vi "输入数据解析.vi"(0 "单个参数补充":dbl, 1 "从板号":dbl=1.0, 2 "主板二维码":string="BNET01", 3 "从板二维码":string="BNET01", 5 "主板引用":refnum<vi>, 7 "从板引用":refnum<vi>, 9 "主板选项":string="三级故障阀值", 11 "枚举":enum16{"主板", "从板"}(ring), 12 "快换":bool caption="快换写入") -> (4 "输出数组":dbl[][](array[numeric]), 6 "数组长度":dbl[](array[numeric]), 8 "循环次数":i32, 10 "命令":u32, 14 "名称":string[](array[string]), 15 "命令序号":u32[](array[numeric]))   [LabVIEW 2013] (continued)
                n1942 = disable-structure shown="启用" {
                  disable-tunnel: [w4961 w4964] -> w4957
                  disable-tunnel: [w4960 w4964] -> w4956
                  disable-tunnel: w4954 -> [w4959 _]
                  frame Disabled {
                    n1943 = Unbundle By Name(w4959) -> ("总电压过低"=w4958:dbl)
                    n1944 = call "输入分辨率计算-EV05.vi"("1字节?"=FALSE, "数值"=w4958, "分辨率"=0.1) -> ("低字节"=w4961:dbl, "高字节1"=w4960:dbl)  [unwired: 2 in, 5 out]
                  }
                  frame Enabled {
                    w4964 = 255 ("高字节1")
                  }
                }
                n1945 = Build Array(w4956, w4957) -> (w4955:i32[])
              }
              frame 2 {
                # "温度过高"
                n1946 = disable-structure shown="启用" {
                  disable-tunnel: [w4971 255 ("高字节1")] -> w4967
                  disable-tunnel: w4965 -> [w4969 _]
                  frame Disabled {
                    n1947 = Unbundle By Name(w4969) -> ("温度过高"=w4968:dbl)
                    n1948 = call "输入分辨率计算-EV05.vi"("1字节?"=TRUE, "数值"=w4968, "偏移量"=-40.0, "分辨率"=1.0) -> ("高字节1"=w4971:dbl)  [unwired: 1 in, 6 out]
                  }
                  frame Enabled {
                  }
                }
                n1949 = Build Array(w4967) -> (w4966:i32[])
              }
              frame 3 {
                # "温度过低"
                n1950 = disable-structure shown="启用" {
                  disable-tunnel: [w4981 255 ("高字节1")] -> w4977
                  disable-tunnel: w4975 -> [w4979 _]
                  frame Disabled {
                    n1951 = Unbundle By Name(w4979) -> ("温度过低"=w4978:dbl)
                    n1952 = call "输入分辨率计算-EV05.vi"("1字节?"=TRUE, "数值"=w4978, "偏移量"=-40.0, "分辨率"=1.0) -> ("高字节1"=w4981:dbl)  [unwired: 1 in, 6 out]
                  }
                  frame Enabled {
                  }
                }
                n1953 = Build Array(w4977) -> (w4976:i32[])
              }
              frame 4 {
                # "整组温度不均衡"
                n1954 = disable-structure shown="启用" {
                  disable-tunnel: [w4991 255 ("高字节1")] -> w4987
                  disable-tunnel: w4985 -> [w4989 _]
                  frame Disabled {
                    n1955 = Unbundle By Name(w4989) -> ("整组温度不均衡"=w4988:dbl)
                    n1956 = call "输入分辨率计算-EV05.vi"("1字节?"=TRUE, "数值"=w4988, "偏移量"=0.0, "分辨率"=1.0) -> ("高字节1"=w4991:dbl)  [unwired: 1 in, 6 out]
                  }
                  frame Enabled {
                  }
                }
                n1957 = Build Array(w4987) -> (w4986:i32[])
              }
              frame 5 {
                # "单组电压不均衡"
                n1958 = disable-structure shown="启用" {
                  disable-tunnel: [w5003 w5006] -> w4998
                  disable-tunnel: [w5001 w5006] -> w4996
                  disable-tunnel: w4995 -> [w5000 _]
                  frame Enabled {
                    n1959 = Unbundle By Name(w5000) -> ("单组电压不均衡"=w4999:dbl)
                    n1960 = call "输入分辨率计算-EV05.vi"("1字节?"=FALSE, "数值"=w4999, "偏移量"=0.0, "分辨率"=0.001) -> ("低字节"=w5001:dbl, "高字节1"=w5003:dbl)  [unwired: 1 in, 5 out]
                  }
                  frame Disabled {
                    w5006 = 255 ("高字节1")
                  }
                }
                n1961 = Build Array(w4998, w4996) -> (w4997:dbl[])
              }
              frame 6 {
                # "整组电压不均衡"
                n1962 = disable-structure shown="启用" {
                  disable-tunnel: [w5015 w5018] -> w5010
                  disable-tunnel: [w5013 w5018] -> w5008
                  disable-tunnel: w5007 -> [w5012 _]
                  frame Disabled {
                    n1963 = Unbundle By Name(w5012) -> ("整组电压不均衡"=w5011:dbl)
                    n1964 = call "输入分辨率计算-EV05.vi"("1字节?"=FALSE, "数值"=w5011, "偏移量"=0.0, "分辨率"=0.001) -> ("低字节"=w5013:dbl, "高字节1"=w5015:dbl)  [unwired: 1 in, 5 out]
                  }
                  frame Enabled {
                    w5018 = 255 ("高字节1")
                  }
                }
                n1965 = Build Array(w5010, w5008) -> (w5009:i32[])
              }
              frame 7 {
                # "单体电压过高"
                n1966 = disable-structure shown="启用" {
                  disable-tunnel: [w5027 w5030] -> w5022
                  disable-tunnel: [w5025 w5030] -> w5020
                  disable-tunnel: w5019 -> [w5024 _]
                  frame Disabled {
                    n1967 = Unbundle By Name(w5024) -> ("单体电压过高"=w5023:dbl)
                    n1968 = call "输入分辨率计算-EV05.vi"("1字节?"=FALSE, "数值"=w5023, "偏移量"=0.0, "分辨率"=0.001) -> ("低字节"=w5025:dbl, "高字节1"=w5027:dbl)  [unwired: 1 in, 5 out]
                  }
                  frame Enabled {
                    w5030 = 255 ("高字节1")
                  }
                }
                n1969 = Build Array(w5022, w5020) -> (w5021:i32[])
              }
              frame 8 {
                # "单体电压过低"
                n1970 = disable-structure shown="启用" {
                  disable-tunnel: [w5039 w5042] -> w5034
                  disable-tunnel: [w5037 w5042] -> w5032
                  disable-tunnel: w5031 -> [w5036 _]
                  frame Disabled {
                    n1971 = Unbundle By Name(w5036) -> ("单体电压过低"=w5035:dbl)
                    n1972 = call "输入分辨率计算-EV05.vi"("1字节?"=FALSE, "数值"=w5035, "偏移量"=0.0, "分辨率"=0.001) -> ("低字节"=w5037:dbl, "高字节1"=w5039:dbl)  [unwired: 1 in, 5 out]
                  }
                  frame Enabled {
                    w5042 = 255 ("高字节1")
                  }
                }
                n1973 = Build Array(w5034, w5032) -> (w5033:i32[])
              }
              frame 9 {
                # "充电电流过高"
                n1974 = disable-structure shown="启用" {
                  disable-tunnel: [w5051 w5054] -> w5046
                  disable-tunnel: [w5049 w5054] -> w5044
                  disable-tunnel: w5043 -> [w5048 _]
                  frame Disabled {
                    n1975 = Unbundle By Name(w5048) -> ("充电电流过高"=w5047:dbl)
                    n1976 = call "输入分辨率计算-EV05.vi"("1字节?"=FALSE, "数值"=w5047, "偏移量"=-3000.0, "分辨率"=0.1) -> ("低字节"=w5049:dbl, "高字节1"=w5051:dbl)  [unwired: 1 in, 5 out]
                  }
                  frame Enabled {
                    w5054 = 255 ("高字节1")
                  }
                }
                n1977 = Build Array(w5046, w5044) -> (w5045:i32[])
              }
              frame 10 {
                # "放电电流过高"
                n1978 = disable-structure shown="启用" {
                  disable-tunnel: [w5063 w5066] -> w5058
                  disable-tunnel: [w5061 w5066] -> w5056
                  disable-tunnel: w5055 -> [w5060 _]
                  frame Disabled {
                    n1979 = Unbundle By Name(w5060) -> ("放电电流过高"=w5059:dbl)
                    n1980 = call "输入分辨率计算-EV05.vi"("1字节?"=FALSE, "数值"=w5059, "偏移量"=-3000.0, "分辨率"=0.1) -> ("低字节"=w5061:dbl, "高字节1"=w5063:dbl)  [unwired: 1 in, 5 out]
                  }
                  frame Enabled {
                    w5066 = 255 ("高字节1")
                  }
                }
                n1981 = Build Array(w5058, w5056) -> (w5057:i32[])
              }
              frame 11 {
                # "单组温度不均衡"
                n1982 = disable-structure shown="启用" {
                  disable-tunnel: [w5073 255 ("高字节1")] -> w5069
                  disable-tunnel: w5067 -> [w5071 _]
                  frame Disabled {
                    n1983 = Unbundle By Name(w5071) -> ("单组温度不均衡"=w5070:dbl)
                    n1984 = call "输入分辨率计算-EV05.vi"("1字节?"=TRUE, "数值"=w5070, "偏移量"=0.0, "分辨率"=1.0) -> ("高字节1"=w5073:dbl)  [unwired: 1 in, 6 out]
                  }
                  frame Enabled {
                  }
                }
                n1985 = Build Array(w5069) -> (w5068:i32[])
              }
              frame 12 {
                # "SOC过高"
                n1986 = Unbundle By Name(w5081) -> ("SOC过高"=w5080:dbl)
                n1987 = call "输入分辨率计算-EV05.vi"("1字节?"=FALSE, "数值"=w5080, "偏移量"=0.0, "分辨率"=0.1) -> ("低字节"=w5082:dbl, "高字节1"=w5083:dbl)  [unwired: 1 in, 5 out]
                n1988 = call "二进制解析-8.6.vi"("索引"=4, "数值"=w5083) -> ("低位子数组"=w5086:i32[])  [unwired: 3 out]
                n1989 = call "二进制解析-8.6.vi"("索引"=4, "数值"=w5082) -> ("低位子数组"=w5078:i32[], "高位子数组"=w5085:i32[])  [unwired: 2 out]
                n1990 = Insert Into Array(array=w5086, new element=w5085) -> (w5084:i32[])  [unwired: 1 in]
                n1991 = call "数值二进制转十进制-8.6.vi"("子数组"=w5084) -> ("十进制数值"=w5079:i32)  [unwired: 4 out]
                n1992 = disable-structure shown="启用" {
                  disable-tunnel: w5079 -> [w5094 _]
                  disable-tunnel: [w5094 255 ("高字节1")] -> w5077
                  disable-tunnel: [w5093 i32[] [] ("低位子数组 23")] -> _
                  disable-tunnel: w5078 -> [w5093 _]
                  frame Disabled {
                  }
                  frame Enabled {
                  }
                }
                n1993 = Build Array(w5077, w5077) -> (w5090:i32[])
              }
              frame 13 {
                # "SOC过低"
                n1994 = Unbundle By Name(w5103) -> ("SOC过低"=w5102:dbl)
                n1995 = call "输入分辨率计算-EV05.vi"("1字节?"=FALSE, "数值"=w5102, "偏移量"=0.0, "分辨率"=0.1) -> ("低字节"=w5100:dbl, "高字节1"=w5101:dbl)  [unwired: 1 in, 5 out]
                n1996 = call "二进制解析-8.6.vi"("索引"=4, "数值"=w5101) -> ("低位子数组"=w5098:i32[])  [unwired: 3 out]
                n1997 = disable-structure shown="启用" {
                  disable-tunnel: w5100 -> [w5110 _]
                  disable-tunnel: [w5110 255 ("高字节1")] -> w5099
                  disable-tunnel: w5098 -> [w5109 _]
                  disable-tunnel: [_ 255 ("高字节1")] -> w5097
                  frame Disabled {
                    (unwired) i32[] [] ("低位子数组 4")
                  }
                  frame Enabled {
                  }
                }
                n1998 = Build Array(w5097, w5099) -> (w5106:i32[])
              }
              frame 14 {
                # "内阻过大"
                n1999 = disable-structure shown="启用" {
                  disable-tunnel: w5115 -> [w5120 _]
                  disable-tunnel: [w5116 255 ("高字节1")] -> w5113
                  frame Disabled {
                    n2000 = Unbundle By Name(w5120) -> ("内阻过大"=w5119:dbl)
                    n2001 = call "输入分辨率计算-EV05.vi"("1字节?"=TRUE, "数值"=w5119, "分辨率"=0.1) -> ("高字节1"=w5116:dbl)  [unwired: 2 in, 6 out]
                  }
                  frame Enabled {
                  }
                }
                n2002 = Build Array(w5113) -> (w5114:i32[])
              }
              frame 15 {
                # "极柱温度过高"
                n2003 = disable-structure shown="启用" {
                  disable-tunnel: w5124 -> [w5130 _]
                  disable-tunnel: [w5126 255 ("高字节1")] -> w5122
                  frame Disabled {
                    n2004 = Unbundle By Name(w5130) -> ("极柱温度过高"=w5129:dbl)
                    n2005 = call "输入分辨率计算-EV05.vi"("1字节?"=TRUE, "数值"=w5129, "偏移量"=-40.0, "分辨率"=1.0) -> ("高字节1"=w5126:dbl)  [unwired: 1 in, 6 out]
                  }
                  frame Enabled {
                  }
                }
                n2006 = Build Array(w5122) -> (w5123:i32[])
              }
              frame 16 {
                # "SOH过低"
                n2007 = disable-structure shown="启用" {
                  disable-tunnel: [w5147 w5155] -> w5134
                  disable-tunnel: w5133 -> [w5144 _]
                  disable-tunnel: [w5136 w5155] -> w5132
                  frame Disabled {
                    n2008 = Unbundle By Name(w5144) -> ("SOH过低"=w5143:dbl)
                    n2009 = call "输入分辨率计算-EV05.vi"("1字节?"=FALSE, "数值"=w5143, "偏移量"=0.0, "分辨率"=0.1) -> ("低字节"=w5145:dbl, "高字节1"=w5146:dbl)  [unwired: 1 in, 5 out]
                    n2010 = call "二进制解析-8.6.vi"("索引"=4, "数值"=w5146) -> ("低位子数组"=w5149:i32[])  [unwired: 3 out]
                    n2011 = call "二进制解析-8.6.vi"("索引"=4, "数值"=w5145) -> ("低位子数组"=w5138:i32[], "高位子数组"=w5148:i32[])  [unwired: 2 out]
                    n2012 = call "二进制解析-8.6.vi"("索引"=4, "数值"=0) -> ("低位子数组"=w5139:i32[])  [unwired: 3 out]
                    n2013 = Insert Into Array(array=w5149, new element=w5148) -> (w5142:i32[])  [unwired: 1 in]
                    n2014 = Insert Into Array(array=w5138, new element=w5139) -> (w5137:i32[])  [unwired: 1 in]
                    n2015 = call "数值二进制转十进制-8.6.vi"("子数组"=w5142) -> ("十进制数值"=w5147:i32)  [unwired: 4 out]
                    n2016 = call "数值二进制转十进制-8.6.vi"("子数组"=w5137) -> ("十进制数值"=w5136:i32)  [unwired: 4 out]
                  }
                  frame Enabled {
                    w5155 = 255 ("高字节1")
                  }
                }
                n2017 = Build Array(w5134, w5132) -> (w5135:i32[])
              }
            }
            n2018 = Insert Into Array(array=w4939, new element=w4940) -> (w4938:dbl[])  [unwired: 1 in]
          }
          n2019 = Build Array(w4935) -> (w4934:dbl[][])
          n2020 = Build Array("三级故障阀值") -> (w4925:string[])
        }
        frame "整组电压不均衡" {
          n2021 = Unbundle By Name(w5161) -> ("一级故障"=w5162:refnum<vi>)
          n2022 = property class="Clust (严格)"(reference=w5162) -> ("Value"=w5160:T4)  [unwired: 1 in, 2 out]
          n2023 = for {
            N: 17 -> [_]
            tunnel: w5160 -> [w5172]
            shift-right: [w5169] -> w5166
            shift-left: dbl[] [] -> [w5170]
            i -> [w5173]
            n2024 = case shown="13" w5173 {
              tunnel: w5172 -> [w5174 w5185 w5196 w5206 w5216 w5226 w5238 w5250 w5262 w5274 w5286 w5298 w5312 w5333 w5344 w5353 w5362]
              tunnel: [w5175 w5186 w5197 w5207 w5217 w5228 w5240 w5252 w5264 w5276 w5288 w5299 w5321 w5336 w5343 w5352 w5364] -> w5171
              frame 0, Default {
                # "总电压过高"
                n2025 = disable-structure shown="启用" {
                  disable-tunnel: [w5181 w5184] -> w5177
                  disable-tunnel: [w5180 w5184] -> w5176
                  disable-tunnel: w5174 -> [w5179 _]
                  frame Disabled {
                    n2026 = Unbundle By Name(w5179) -> ("总电压过高"=w5178:dbl)
                    n2027 = call "输入分辨率计算-EV05.vi"("1字节?"=FALSE, "数值"=w5178, "分辨率"=0.1) -> ("低字节"=w5181:dbl, "高字节1"=w5180:dbl)  [unwired: 2 in, 5 out]
                  }
                  frame Enabled {
                    w5184 = 255 ("高字节1")
                  }
                }
                n2028 = Build Array(w5176, w5177) -> (w5175:i32[])
              }
              frame 1 {
                # "总电压过低"
                n2029 = disable-structure shown="启用" {
                  disable-tunnel: [w5192 w5195] -> w5188
                  disable-tunnel: [w5191 w5195] -> w5187
                  disable-tunnel: w5185 -> [w5190 _]
                  frame Disabled {
                    n2030 = Unbundle By Name(w5190) -> ("总电压过低"=w5189:dbl)
                    n2031 = call "输入分辨率计算-EV05.vi"("1字节?"=FALSE, "数值"=w5189, "分辨率"=0.1) -> ("低字节"=w5192:dbl, "高字节1"=w5191:dbl)  [unwired: 2 in, 5 out]
                  }
                  frame Enabled {
                    w5195 = 255 ("高字节1")
                  }
                }
                n2032 = Build Array(w5187, w5188) -> (w5186:i32[])
              }
              frame 2 {
                # "温度过高"
                n2033 = disable-structure shown="启用" {
                  disable-tunnel: [w5202 255 ("高字节1")] -> w5198
                  disable-tunnel: w5196 -> [w5200 _]
                  frame Disabled {
                    n2034 = Unbundle By Name(w5200) -> ("温度过高"=w5199:dbl)
                    n2035 = call "输入分辨率计算-EV05.vi"("1字节?"=TRUE, "数值"=w5199, "偏移量"=-40.0, "分辨率"=1.0) -> ("高字节1"=w5202:dbl)  [unwired: 1 in, 6 out]
                  }
                  frame Enabled {
                  }
                }
                n2036 = Build Array(w5198) -> (w5197:i32[])
              }
              frame 3 {
                # "温度过低"
                n2037 = disable-structure shown="启用" {
                  disable-tunnel: [w5212 255 ("高字节1")] -> w5208
                  disable-tunnel: w5206 -> [w5210 _]
                  frame Disabled {
                    n2038 = Unbundle By Name(w5210) -> ("温度过低"=w5209:dbl)
                    n2039 = call "输入分辨率计算-EV05.vi"("1字节?"=TRUE, "数值"=w5209, "偏移量"=-40.0, "分辨率"=1.0) -> ("高字节1"=w5212:dbl)  [unwired: 1 in, 6 out]
                  }
                  frame Enabled {
                  }
                }
                n2040 = Build Array(w5208) -> (w5207:i32[])
              }
              frame 4 {
                # "整组温度不均衡"
                n2041 = disable-structure shown="启用" {
                  disable-tunnel: [w5222 255 ("高字节1")] -> w5218
                  disable-tunnel: w5216 -> [w5220 _]
                  frame Disabled {
                    n2042 = Unbundle By Name(w5220) -> ("整组温度不均衡"=w5219:dbl)
                    n2043 = call "输入分辨率计算-EV05.vi"("1字节?"=TRUE, "数值"=w5219, "偏移量"=0.0, "分辨率"=1.0) -> ("高字节1"=w5222:dbl)  [unwired: 1 in, 6 out]
                  }
                  frame Enabled {
                  }
                }
                n2044 = Build Array(w5218) -> (w5217:i32[])
              }
              frame 5 {
                # "单组电压不均衡"
                n2045 = disable-structure shown="启用" {
                  disable-tunnel: [w5234 w5237] -> w5229
                  disable-tunnel: [w5232 w5237] -> w5227
                  disable-tunnel: w5226 -> [w5231 _]
                  frame Disabled {
                    n2046 = Unbundle By Name(w5231) -> ("单组电压不均衡"=w5230:dbl)
                    n2047 = call "输入分辨率计算-EV05.vi"("1字节?"=FALSE, "数值"=w5230, "偏移量"=0.0, "分辨率"=0.001) -> ("低字节"=w5232:dbl, "高字节1"=w5234:dbl)  [unwired: 1 in, 5 out]
                  }
                  frame Enabled {
                    w5237 = 255 ("高字节1")
                  }
                }
                n2048 = Build Array(w5229, w5227) -> (w5228:i32[])
              }
              frame 6 {
                # "整组电压不均衡"
                n2049 = disable-structure shown="启用" {
                  disable-tunnel: [w5246 w5249] -> w5241
                  disable-tunnel: [w5244 w5249] -> w5239
                  disable-tunnel: w5238 -> [w5243 _]
                  frame Enabled {
                    n2050 = Unbundle By Name(w5243) -> ("整组电压不均衡"=w5242:dbl)
                    n2051 = call "输入分辨率计算-EV05.vi"("1字节?"=FALSE, "数值"=w5242, "偏移量"=0.0, "分辨率"=0.001) -> ("低字节"=w5244:dbl, "高字节1"=w5246:dbl)  [unwired: 1 in, 5 out]
                  }
                  frame Disabled {
                    w5249 = 255 ("高字节1")
                  }
                }
                n2052 = Build Array(w5241, w5239) -> (w5240:dbl[])
              }
              frame 7 {
                # "单体电压过高"
                n2053 = disable-structure shown="启用" {
                  disable-tunnel: [w5258 w5261] -> w5253
                  disable-tunnel: [w5256 w5261] -> w5251
                  disable-tunnel: w5250 -> [w5255 _]
                  frame Disabled {
                    n2054 = Unbundle By Name(w5255) -> ("单体电压过高"=w5254:dbl)
                    n2055 = call "输入分辨率计算-EV05.vi"("1字节?"=FALSE, "数值"=w5254, "偏移量"=0.0, "分辨率"=0.001) -> ("低字节"=w5256:dbl, "高字节1"=w5258:dbl)  [unwired: 1 in, 5 out]
                  }
                  frame Enabled {
                    w5261 = 255 ("高字节1")
                  }
                }
                n2056 = Build Array(w5253, w5251) -> (w5252:i32[])
              }
              frame 8 {
                # "单体电压过低"
                n2057 = disable-structure shown="启用" {
                  disable-tunnel: [w5270 w5273] -> w5265
                  disable-tunnel: [w5268 w5273] -> w5263
                  disable-tunnel: w5262 -> [w5267 _]
                  frame Disabled {
                    n2058 = Unbundle By Name(w5267) -> ("单体电压过低"=w5266:dbl)
                    n2059 = call "输入分辨率计算-EV05.vi"("1字节?"=FALSE, "数值"=w5266, "偏移量"=0.0, "分辨率"=0.001) -> ("低字节"=w5268:dbl, "高字节1"=w5270:dbl)  [unwired: 1 in, 5 out]
                  }
                  frame Enabled {
                    w5273 = 255 ("高字节1")
                  }
                }
                n2060 = Build Array(w5265, w5263) -> (w5264:i32[])
              }
              frame 9 {
                # "充电电流过高"
                n2061 = disable-structure shown="启用" {
                  disable-tunnel: [w5282 w5285] -> w5277
                  disable-tunnel: [w5280 w5285] -> w5275
                  disable-tunnel: w5274 -> [w5279 _]
                  frame Disabled {
                    n2062 = Unbundle By Name(w5279) -> ("充电电流过高"=w5278:dbl)
                    n2063 = call "输入分辨率计算-EV05.vi"("1字节?"=FALSE, "数值"=w5278, "偏移量"=-3000.0, "分辨率"=0.1) -> ("低字节"=w5280:dbl, "高字节1"=w5282:dbl)  [unwired: 1 in, 5 out]
                  }
                  frame Enabled {
                    w5285 = 255 ("高字节1")
                  }
                }
                n2064 = Build Array(w5277, w5275) -> (w5276:i32[])
              }
              frame 10 {
                # "放电电流过高"
                n2065 = disable-structure shown="启用" {
                  disable-tunnel: [w5294 w5297] -> w5289
                  disable-tunnel: [w5292 w5297] -> w5287
                  disable-tunnel: w5286 -> [w5291 _]
                  frame Disabled {
                    n2066 = Unbundle By Name(w5291) -> ("放电电流过高"=w5290:dbl)
                    n2067 = call "输入分辨率计算-EV05.vi"("1字节?"=FALSE, "数值"=w5290, "偏移量"=-3000.0, "分辨率"=0.1) -> ("低字节"=w5292:dbl, "高字节1"=w5294:dbl)  [unwired: 1 in, 5 out]
                  }
                  frame Enabled {
                    w5297 = 255 ("高字节1")
                  }
                }
                n2068 = Build Array(w5289, w5287) -> (w5288:i32[])
              }
              frame 11 {
                # "单组温度不均衡"
                n2069 = disable-structure shown="启用" {
                  disable-tunnel: [w5304 255 ("高字节1")] -> w5300
                  disable-tunnel: w5298 -> [w5302 _]
                  frame Disabled {
                    n2070 = Unbundle By Name(w5302) -> ("单组温度不均衡"=w5301:dbl)
                    n2071 = call "输入分辨率计算-EV05.vi"("1字节?"=TRUE, "数值"=w5301, "偏移量"=0.0, "分辨率"=1.0) -> ("高字节1"=w5304:dbl)  [unwired: 1 in, 6 out]
                  }
                  frame Enabled {
                  }
                }
                n2072 = Build Array(w5300) -> (w5299:i32[])
              }
              frame 12 {
                # "SOC过高"
                n2073 = Unbundle By Name(w5312) -> ("SOC过高"=w5311:dbl)
                n2074 = call "输入分辨率计算-EV05.vi"("1字节?"=FALSE, "数值"=w5311, "偏移量"=0.0, "分辨率"=0.1) -> ("低字节"=w5313:dbl, "高字节1"=w5314:dbl)  [unwired: 1 in, 5 out]
                n2075 = call "二进制解析-8.6.vi"("索引"=4, "数值"=w5314) -> ("低位子数组"=w5317:i32[])  [unwired: 3 out]
                n2076 = call "二进制解析-8.6.vi"("索引"=4, "数值"=w5313) -> ("低位子数组"=w5309:i32[], "高位子数组"=w5316:i32[])  [unwired: 2 out]
                n2077 = Insert Into Array(array=w5317, new element=w5316) -> (w5315:i32[])  [unwired: 1 in]
                n2078 = call "数值二进制转十进制-8.6.vi"("子数组"=w5315) -> ("十进制数值"=w5310:i32)  [unwired: 4 out]
                n2079 = disable-structure shown="启用" {
                  disable-tunnel: w5310 -> [w5325 _]
                  disable-tunnel: [w5325 255 ("高字节1")] -> w5308
                  disable-tunnel: [w5324 i32[] [] ("低位子数组 24")] -> _
                  disable-tunnel: w5309 -> [w5324 _]
                  frame Disabled {
                  }
                  frame Enabled {
                  }
                }
                n2080 = Build Array(w5308, w5308) -> (w5321:i32[])
              }
              frame 13 {
                # "SOC过低"
                n2081 = Unbundle By Name(w5333) -> ("SOC过低"=w5332:dbl)
                n2082 = call "输入分辨率计算-EV05.vi"("1字节?"=FALSE, "数值"=w5332, "偏移量"=0.0, "分辨率"=0.1) -> ("低字节"=w5330:dbl, "高字节1"=w5331:dbl)  [unwired: 1 in, 5 out]
                n2083 = call "二进制解析-8.6.vi"("索引"=4, "数值"=w5331) -> ("低位子数组"=w5329:i32[])  [unwired: 3 out]
                n2084 = disable-structure shown="启用" {
                  disable-tunnel: w5330 -> [w5340 _]
                  disable-tunnel: [w5340 255 ("高字节1")] -> w5328
                  disable-tunnel: w5329 -> [w5339 _]
                  frame Disabled {
                    (unwired) i32[] [] ("低位子数组 4")
                  }
                  frame Enabled {
                  }
                }
                n2085 = Build Array(w5328, w5328) -> (w5336:i32[])
              }
              frame 14 {
                # "内阻过大"
                n2086 = disable-structure shown="启用" {
                  disable-tunnel: w5344 -> [w5349 _]
                  disable-tunnel: [w5345 255 ("高字节1")] -> w5342
                  frame Disabled {
                    n2087 = Unbundle By Name(w5349) -> ("内阻过大"=w5348:dbl)
                    n2088 = call "输入分辨率计算-EV05.vi"("1字节?"=TRUE, "数值"=w5348, "分辨率"=0.1) -> ("高字节1"=w5345:dbl)  [unwired: 2 in, 6 out]
                  }
                  frame Enabled {
                  }
                }
                n2089 = Build Array(w5342) -> (w5343:i32[])
              }
              frame 15 {
                # "极柱温度过高"
                n2090 = disable-structure shown="启用" {
                  disable-tunnel: w5353 -> [w5359 _]
                  disable-tunnel: [w5355 255 ("高字节1")] -> w5351
                  frame Disabled {
                    n2091 = Unbundle By Name(w5359) -> ("极柱温度过高"=w5358:dbl)
                    n2092 = call "输入分辨率计算-EV05.vi"("1字节?"=TRUE, "数值"=w5358, "偏移量"=-40.0, "分辨率"=1.0) -> ("高字节1"=w5355:dbl)  [unwired: 1 in, 6 out]
                  }
                  frame Enabled {
                  }
                }
                n2093 = Build Array(w5351) -> (w5352:i32[])
              }
              frame 16 {
                # "SOH过低"
                n2094 = disable-structure shown="启用" {
                  disable-tunnel: [w5376 w5384] -> w5363
                  disable-tunnel: w5362 -> [w5373 _]
                  disable-tunnel: [w5365 w5384] -> w5361
                  frame Disabled {
                    n2095 = Unbundle By Name(w5373) -> ("SOH过低"=w5372:dbl)
                    n2096 = call "输入分辨率计算-EV05.vi"("1字节?"=FALSE, "数值"=w5372, "偏移量"=0.0, "分辨率"=0.1) -> ("低字节"=w5374:dbl, "高字节1"=w5375:dbl)  [unwired: 1 in, 5 out]
                    n2097 = call "二进制解析-8.6.vi"("索引"=4, "数值"=w5375) -> ("低位子数组"=w5378:i32[])  [unwired: 3 out]
                    n2098 = call "二进制解析-8.6.vi"("索引"=4, "数值"=w5374) -> ("低位子数组"=w5367:i32[], "高位子数组"=w5377:i32[])  [unwired: 2 out]
                    n2099 = call "二进制解析-8.6.vi"("索引"=4, "数值"=0) -> ("低位子数组"=w5368:i32[])  [unwired: 3 out]
                    n2100 = Insert Into Array(array=w5378, new element=w5377) -> (w5371:i32[])  [unwired: 1 in]
                    n2101 = Insert Into Array(array=w5367, new element=w5368) -> (w5366:i32[])  [unwired: 1 in]
                    n2102 = call "数值二进制转十进制-8.6.vi"("子数组"=w5371) -> ("十进制数值"=w5376:i32)  [unwired: 4 out]
                    n2103 = call "数值二进制转十进制-8.6.vi"("子数组"=w5366) -> ("十进制数值"=w5365:i32)  [unwired: 4 out]
                  }
                  frame Enabled {
                    w5384 = 255 ("高字节1")
                  }
                }
                n2104 = Build Array(w5363, w5361) -> (w5364:i32[])
              }
            }
            n2105 = Insert Into Array(array=w5170, new element=w5171) -> (w5169:dbl[])  [unwired: 1 in]
          }
          n2106 = Build Array(w5166) -> (w5165:dbl[][])
          n2107 = Build Array("一级故障阀值") -> (w5156:string[])
        }
        frame "整组电压不均衡(2)" {
          n2108 = Unbundle By Name(w5390) -> ("一级故障 2"=w5391:refnum<vi>)
          n2109 = property class="Clust (严格)"(reference=w5391) -> ("Value"=w5389:T4)  [unwired: 1 in, 2 out]
          n2110 = for {
            N: 17 -> [_]
            tunnel: w5389 -> [w5401]
            shift-right: [w5398] -> w5395
            shift-left: dbl[] [] -> [w5399]
            i -> [w5402]
            n2111 = case shown="13" w5402 {
              tunnel: w5401 -> [w5403 w5414 w5425 w5435 w5445 w5455 w5467 w5479 w5491 w5503 w5515 w5527 w5541 w5562 w5573 w5582 w5591]
              tunnel: [w5404 w5415 w5426 w5436 w5446 w5457 w5469 w5481 w5493 w5505 w5517 w5528 w5550 w5565 w5572 w5581 w5593] -> w5400
              frame 0, Default {
                # "总电压过高"
                n2112 = disable-structure shown="启用" {
                  disable-tunnel: [w5410 w5413] -> w5406
                  disable-tunnel: [w5409 w5413] -> w5405
                  disable-tunnel: w5403 -> [w5408 _]
                  frame Disabled {
                    n2113 = Unbundle By Name(w5408) -> ("总电压过高"=w5407:dbl)
                    n2114 = call "输入分辨率计算-EV05.vi"("1字节?"=FALSE, "数值"=w5407, "分辨率"=0.1) -> ("低字节"=w5410:dbl, "高字节1"=w5409:dbl)  [unwired: 2 in, 5 out]
                  }
                  frame Enabled {
                    w5413 = 255 ("高字节1")
                  }
                }
                n2115 = Build Array(w5405, w5406) -> (w5404:i32[])
              }
              frame 1 {
                # "总电压过低"
                n2116 = disable-structure shown="启用" {
                  disable-tunnel: [w5421 w5424] -> w5417
                  disable-tunnel: [w5420 w5424] -> w5416
                  disable-tunnel: w5414 -> [w5419 _]
                  frame Disabled {
                    n2117 = Unbundle By Name(w5419) -> ("总电压过低"=w5418:dbl)
                    n2118 = call "输入分辨率计算-EV05.vi"("1字节?"=FALSE, "数值"=w5418, "分辨率"=0.1) -> ("低字节"=w5421:dbl, "高字节1"=w5420:dbl)  [unwired: 2 in, 5 out]
                  }
                  frame Enabled {
                    w5424 = 255 ("高字节1")
                  }
                }
                n2119 = Build Array(w5416, w5417) -> (w5415:i32[])
              }
              frame 2 {
                # "温度过高"
                n2120 = disable-structure shown="启用" {
                  disable-tunnel: [w5431 255 ("高字节1")] -> w5427
                  disable-tunnel: w5425 -> [w5429 _]
                  frame Disabled {
                    n2121 = Unbundle By Name(w5429) -> ("温度过高"=w5428:dbl)
                    n2122 = call "输入分辨率计算-EV05.vi"("1字节?"=TRUE, "数值"=w5428, "偏移量"=-40.0, "分辨率"=1.0) -> ("高字节1"=w5431:dbl)  [unwired: 1 in, 6 out]
                  }
                  frame Enabled {
                  }
                }
                n2123 = Build Array(w5427) -> (w5426:i32[])
              }
              frame 3 {
                # "温度过低"
                n2124 = disable-structure shown="启用" {
                  disable-tunnel: [w5441 255 ("高字节1")] -> w5437
                  disable-tunnel: w5435 -> [w5439 _]
                  frame Disabled {
                    n2125 = Unbundle By Name(w5439) -> ("温度过低"=w5438:dbl)
                    n2126 = call "输入分辨率计算-EV05.vi"("1字节?"=TRUE, "数值"=w5438, "偏移量"=-40.0, "分辨率"=1.0) -> ("高字节1"=w5441:dbl)  [unwired: 1 in, 6 out]
                  }
                  frame Enabled {
                  }
                }
                n2127 = Build Array(w5437) -> (w5436:i32[])
              }
              frame 4 {
                # "整组温度不均衡"
                n2128 = disable-structure shown="启用" {
                  disable-tunnel: [w5451 255 ("高字节1")] -> w5447
                  disable-tunnel: w5445 -> [w5449 _]
                  frame Disabled {
                    n2129 = Unbundle By Name(w5449) -> ("整组温度不均衡"=w5448:dbl)
                    n2130 = call "输入分辨率计算-EV05.vi"("1字节?"=TRUE, "数值"=w5448, "偏移量"=0.0, "分辨率"=1.0) -> ("高字节1"=w5451:dbl)  [unwired: 1 in, 6 out]
                  }
                  frame Enabled {
                  }
                }
                n2131 = Build Array(w5447) -> (w5446:i32[])
              }
              frame 5 {
                # "单组电压不均衡"
                n2132 = disable-structure shown="启用" {
                  disable-tunnel: [w5463 w5466] -> w5458
                  disable-tunnel: [w5461 w5466] -> w5456
                  disable-tunnel: w5455 -> [w5460 _]
                  frame Disabled {
                    n2133 = Unbundle By Name(w5460) -> ("单组电压不均衡"=w5459:dbl)
                    n2134 = call "输入分辨率计算-EV05.vi"("1字节?"=FALSE, "数值"=w5459, "偏移量"=0.0, "分辨率"=0.001) -> ("低字节"=w5461:dbl, "高字节1"=w5463:dbl)  [unwired: 1 in, 5 out]
                  }
                  frame Enabled {
                    w5466 = 255 ("高字节1")
                  }
                }
                n2135 = Build Array(w5458, w5456) -> (w5457:i32[])
              }
              frame 6 {
                # "整组电压不均衡"
                n2136 = disable-structure shown="启用" {
                  disable-tunnel: [w5475 w5478] -> w5470
                  disable-tunnel: [w5473 w5478] -> w5468
                  disable-tunnel: w5467 -> [w5472 _]
                  frame Enabled {
                    n2137 = Unbundle By Name(w5472) -> ("整组电压不均衡"=w5471:dbl)
                    n2138 = call "输入分辨率计算-EV05.vi"("1字节?"=FALSE, "数值"=w5471, "偏移量"=0.0, "分辨率"=0.001) -> ("低字节"=w5473:dbl, "高字节1"=w5475:dbl)  [unwired: 1 in, 5 out]
                  }
                  frame Disabled {
                    w5478 = 255 ("高字节1")
                  }
                }
                n2139 = Build Array(w5470, w5468) -> (w5469:dbl[])
              }
              frame 7 {
                # "单体电压过高"
                n2140 = disable-structure shown="启用" {
                  disable-tunnel: [w5487 w5490] -> w5482
                  disable-tunnel: [w5485 w5490] -> w5480
                  disable-tunnel: w5479 -> [w5484 _]
                  frame Disabled {
                    n2141 = Unbundle By Name(w5484) -> ("单体电压过高"=w5483:dbl)
                    n2142 = call "输入分辨率计算-EV05.vi"("1字节?"=FALSE, "数值"=w5483, "偏移量"=0.0, "分辨率"=0.001) -> ("低字节"=w5485:dbl, "高字节1"=w5487:dbl)  [unwired: 1 in, 5 out]
                  }
                  frame Enabled {
                    w5490 = 255 ("高字节1")
                  }
                }
                n2143 = Build Array(w5482, w5480) -> (w5481:i32[])
              }
              frame 8 {
                # "单体电压过低"
                n2144 = disable-structure shown="启用" {
                  disable-tunnel: [w5499 w5502] -> w5494
                  disable-tunnel: [w5497 w5502] -> w5492
                  disable-tunnel: w5491 -> [w5496 _]
                  frame Disabled {
                    n2145 = Unbundle By Name(w5496) -> ("单体电压过低"=w5495:dbl)
                    n2146 = call "输入分辨率计算-EV05.vi"("1字节?"=FALSE, "数值"=w5495, "偏移量"=0.0, "分辨率"=0.001) -> ("低字节"=w5497:dbl, "高字节1"=w5499:dbl)  [unwired: 1 in, 5 out]
                  }
                  frame Enabled {
                    w5502 = 255 ("高字节1")
                  }
                }
                n2147 = Build Array(w5494, w5492) -> (w5493:i32[])
              }
              frame 9 {
                # "充电电流过高"
                n2148 = disable-structure shown="启用" {
                  disable-tunnel: [w5511 w5514] -> w5506
                  disable-tunnel: [w5509 w5514] -> w5504
                  disable-tunnel: w5503 -> [w5508 _]
                  frame Disabled {
                    n2149 = Unbundle By Name(w5508) -> ("充电电流过高"=w5507:dbl)
                    n2150 = call "输入分辨率计算-EV05.vi"("1字节?"=FALSE, "数值"=w5507, "偏移量"=-3000.0, "分辨率"=0.1) -> ("低字节"=w5509:dbl, "高字节1"=w5511:dbl)  [unwired: 1 in, 5 out]
                  }
                  frame Enabled {
                    w5514 = 255 ("高字节1")
                  }
                }
                n2151 = Build Array(w5506, w5504) -> (w5505:i32[])
              }
              frame 10 {
                # "放电电流过高"
                n2152 = disable-structure shown="启用" {
                  disable-tunnel: [w5523 w5526] -> w5518
                  disable-tunnel: [w5521 w5526] -> w5516
                  disable-tunnel: w5515 -> [w5520 _]
                  frame Disabled {
                    n2153 = Unbundle By Name(w5520) -> ("放电电流过高"=w5519:dbl)
                    n2154 = call "输入分辨率计算-EV05.vi"("1字节?"=FALSE, "数值"=w5519, "偏移量"=-3000.0, "分辨率"=0.1) -> ("低字节"=w5521:dbl, "高字节1"=w5523:dbl)  [unwired: 1 in, 5 out]
                  }
                  frame Enabled {
                    w5526 = 255 ("高字节1")
                  }
                }
                n2155 = Build Array(w5518, w5516) -> (w5517:i32[])
              }
              frame 11 {
                # "单组温度不均衡"
                n2156 = disable-structure shown="启用" {
                  disable-tunnel: [w5533 255 ("高字节1")] -> w5529
                  disable-tunnel: w5527 -> [w5531 _]
                  frame Disabled {
                    n2157 = Unbundle By Name(w5531) -> ("单组温度不均衡"=w5530:dbl)
                    n2158 = call "输入分辨率计算-EV05.vi"("1字节?"=TRUE, "数值"=w5530, "偏移量"=0.0, "分辨率"=1.0) -> ("高字节1"=w5533:dbl)  [unwired: 1 in, 6 out]
                  }
                  frame Enabled {
                  }
                }
                n2159 = Build Array(w5529) -> (w5528:i32[])
              }
              frame 12 {
                # "SOC过高"
                n2160 = Unbundle By Name(w5541) -> ("SOC过高"=w5540:dbl)
                n2161 = call "输入分辨率计算-EV05.vi"("1字节?"=FALSE, "数值"=w5540, "偏移量"=0.0, "分辨率"=0.1) -> ("低字节"=w5542:dbl, "高字节1"=w5543:dbl)  [unwired: 1 in, 5 out]
                n2162 = call "二进制解析-8.6.vi"("索引"=4, "数值"=w5543) -> ("低位子数组"=w5546:i32[])  [unwired: 3 out]
                n2163 = call "二进制解析-8.6.vi"("索引"=4, "数值"=w5542) -> ("低位子数组"=w5538:i32[], "高位子数组"=w5545:i32[])  [unwired: 2 out]
                n2164 = Insert Into Array(array=w5546, new element=w5545) -> (w5544:i32[])  [unwired: 1 in]
                n2165 = call "数值二进制转十进制-8.6.vi"("子数组"=w5544) -> ("十进制数值"=w5539:i32)  [unwired: 4 out]
                n2166 = disable-structure shown="启用" {
                  disable-tunnel: w5539 -> [w5554 _]
                  disable-tunnel: [w5554 255 ("高字节1")] -> w5537
                  disable-tunnel: [w5553 i32[] [] ("低位子数组 24")] -> _
                  disable-tunnel: w5538 -> [w5553 _]
                  frame Disabled {
                  }
                  frame Enabled {
                  }
                }
                n2167 = Build Array(w5537, w5537) -> (w5550:i32[])
              }
              frame 13 {
                # "SOC过低"
                n2168 = Unbundle By Name(w5562) -> ("SOC过低"=w5561:dbl)
                n2169 = call "输入分辨率计算-EV05.vi"("1字节?"=FALSE, "数值"=w5561, "偏移量"=0.0, "分辨率"=0.1) -> ("低字节"=w5559:dbl, "高字节1"=w5560:dbl)  [unwired: 1 in, 5 out]
                n2170 = call "二进制解析-8.6.vi"("索引"=4, "数值"=w5560) -> ("低位子数组"=w5558:i32[])  [unwired: 3 out]
                n2171 = disable-structure shown="启用" {
                  disable-tunnel: w5559 -> [w5569 _]
                  disable-tunnel: [w5569 255 ("高字节1")] -> w5557
                  disable-tunnel: w5558 -> [w5568 _]
                  frame Disabled {
                    (unwired) i32[] [] ("低位子数组 4")
                  }
                  frame Enabled {
                  }
                }
                n2172 = Build Array(w5557, w5557) -> (w5565:i32[])
              }
              frame 14 {
                # "内阻过大"
                n2173 = disable-structure shown="启用" {
                  disable-tunnel: w5573 -> [w5578 _]
                  disable-tunnel: [w5574 255 ("高字节1")] -> w5571
                  frame Disabled {
                    n2174 = Unbundle By Name(w5578) -> ("内阻过大"=w5577:dbl)
                    n2175 = call "输入分辨率计算-EV05.vi"("1字节?"=TRUE, "数值"=w5577, "分辨率"=0.1) -> ("高字节1"=w5574:dbl)  [unwired: 2 in, 6 out]
                  }
                  frame Enabled {
                  }
                }
                n2176 = Build Array(w5571) -> (w5572:i32[])
              }
              frame 15 {
                # "极柱温度过高"
                n2177 = disable-structure shown="启用" {
                  disable-tunnel: w5582 -> [w5588 _]
                  disable-tunnel: [w5584 255 ("高字节1")] -> w5580
                  frame Disabled {
                    n2178 = Unbundle By Name(w5588) -> ("极柱温度过高"=w5587:dbl)
                    n2179 = call "输入分辨率计算-EV05.vi"("1字节?"=TRUE, "数值"=w5587, "偏移量"=-40.0, "分辨率"=1.0) -> ("高字节1"=w5584:dbl)  [unwired: 1 in, 6 out]
                  }
                  frame Enabled {
                  }
                }
                n2180 = Build Array(w5580) -> (w5581:i32[])
              }
              frame 16 {
                # "SOH过低"
                n2181 = disable-structure shown="启用" {
                  disable-tunnel: [w5605 w5613] -> w5592
                  disable-tunnel: w5591 -> [w5602 _]
                  disable-tunnel: [w5594 w5613] -> w5590
                  frame Disabled {
                    n2182 = Unbundle By Name(w5602) -> ("SOH过低"=w5601:dbl)
                    n2183 = call "输入分辨率计算-EV05.vi"("1字节?"=FALSE, "数值"=w5601, "偏移量"=0.0, "分辨率"=0.1) -> ("低字节"=w5603:dbl, "高字节1"=w5604:dbl)  [unwired: 1 in, 5 out]
                    n2184 = call "二进制解析-8.6.vi"("索引"=4, "数值"=w5604) -> ("低位子数组"=w5607:i32[])  [unwired: 3 out]
                    n2185 = call "二进制解析-8.6.vi"("索引"=4, "数值"=w5603) -> ("低位子数组"=w5596:i32[], "高位子数组"=w5606:i32[])  [unwired: 2 out]
                    n2186 = call "二进制解析-8.6.vi"("索引"=4, "数值"=0) -> ("低位子数组"=w5597:i32[])  [unwired: 3 out]
                    n2187 = Insert Into Array(array=w5607, new element=w5606) -> (w5600:i32[])  [unwired: 1 in]
                    n2188 = Insert Into Array(array=w5596, new element=w5597) -> (w5595:i32[])  [unwired: 1 in]
                    n2189 = call "数值二进制转十进制-8.6.vi"("子数组"=w5600) -> ("十进制数值"=w5605:i32)  [unwired: 4 out]
                    n2190 = call "数值二进制转十进制-8.6.vi"("子数组"=w5595) -> ("十进制数值"=w5594:i32)  [unwired: 4 out]
                  }
                  frame Enabled {
                    w5613 = 255 ("高字节1")
                  }
                }
                n2191 = Build Array(w5592, w5590) -> (w5593:i32[])
              }
            }
            n2192 = Insert Into Array(array=w5399, new element=w5400) -> (w5398:dbl[])  [unwired: 1 in]
          }
          n2193 = Build Array(w5395) -> (w5394:dbl[][])
          n2194 = Build Array("二级故障阀值") -> (w5385:string[])
        }
        frame "整组电压不均衡(3)" {
          n2195 = Unbundle By Name(w5619) -> ("一级故障 3"=w5620:refnum<vi>)
          n2196 = property class="Clust (严格)"(reference=w5620) -> ("Value"=w5618:T4)  [unwired: 1 in, 2 out]
          n2197 = for {
            N: 17 -> [_]
            tunnel: w5618 -> [w5630]
            shift-right: [w5627] -> w5624
            shift-left: dbl[] [] -> [w5628]
            i -> [w5631]
            n2198 = case shown="13" w5631 {
              tunnel: w5630 -> [w5632 w5643 w5654 w5664 w5674 w5684 w5696 w5708 w5720 w5732 w5744 w5756 w5770 w5791 w5802 w5811 w5820]
              tunnel: [w5633 w5644 w5655 w5665 w5675 w5686 w5698 w5710 w5722 w5734 w5746 w5757 w5779 w5794 w5801 w5810 w5822] -> w5629
              frame 0, Default {
                # "总电压过高"
                n2199 = disable-structure shown="启用" {
                  disable-tunnel: [w5639 w5642] -> w5635
                  disable-tunnel: [w5638 w5642] -> w5634
                  disable-tunnel: w5632 -> [w5637 _]
                  frame Disabled {
                    n2200 = Unbundle By Name(w5637) -> ("总电压过高"=w5636:dbl)
                    n2201 = call "输入分辨率计算-EV05.vi"("1字节?"=FALSE, "数值"=w5636, "分辨率"=0.1) -> ("低字节"=w5639:dbl, "高字节1"=w5638:dbl)  [unwired: 2 in, 5 out]
                  }
                  frame Enabled {
                    w5642 = 255 ("高字节1")
                  }
                }
                n2202 = Build Array(w5634, w5635) -> (w5633:i32[])
              }
              frame 1 {
                # "总电压过低"
                n2203 = disable-structure shown="启用" {
                  disable-tunnel: [w5650 w5653] -> w5646
                  disable-tunnel: [w5649 w5653] -> w5645
                  disable-tunnel: w5643 -> [w5648 _]
                  frame Disabled {
                    n2204 = Unbundle By Name(w5648) -> ("总电压过低"=w5647:dbl)
                    n2205 = call "输入分辨率计算-EV05.vi"("1字节?"=FALSE, "数值"=w5647, "分辨率"=0.1) -> ("低字节"=w5650:dbl, "高字节1"=w5649:dbl)  [unwired: 2 in, 5 out]
                  }
                  frame Enabled {
                    w5653 = 255 ("高字节1")
                  }
                }
                n2206 = Build Array(w5645, w5646) -> (w5644:i32[])
              }
              frame 2 {
                # "温度过高"
                n2207 = disable-structure shown="启用" {
                  disable-tunnel: [w5660 255 ("高字节1")] -> w5656
                  disable-tunnel: w5654 -> [w5658 _]
                  frame Disabled {
                    n2208 = Unbundle By Name(w5658) -> ("温度过高"=w5657:dbl)
                    n2209 = call "输入分辨率计算-EV05.vi"("1字节?"=TRUE, "数值"=w5657, "偏移量"=-40.0, "分辨率"=1.0) -> ("高字节1"=w5660:dbl)  [unwired: 1 in, 6 out]
                  }
                  frame Enabled {
                  }
                }
                n2210 = Build Array(w5656) -> (w5655:i32[])
              }
              frame 3 {
                # "温度过低"
                n2211 = disable-structure shown="启用" {
                  disable-tunnel: [w5670 255 ("高字节1")] -> w5666
                  disable-tunnel: w5664 -> [w5668 _]
                  frame Disabled {
                    n2212 = Unbundle By Name(w5668) -> ("温度过低"=w5667:dbl)
                    n2213 = call "输入分辨率计算-EV05.vi"("1字节?"=TRUE, "数值"=w5667, "偏移量"=-40.0, "分辨率"=1.0) -> ("高字节1"=w5670:dbl)  [unwired: 1 in, 6 out]
                  }
                  frame Enabled {
                  }
                }
                n2214 = Build Array(w5666) -> (w5665:i32[])
              }
              frame 4 {
                # "整组温度不均衡"
                n2215 = disable-structure shown="启用" {
                  disable-tunnel: [w5680 255 ("高字节1")] -> w5676
                  disable-tunnel: w5674 -> [w5678 _]
                  frame Disabled {
                    n2216 = Unbundle By Name(w5678) -> ("整组温度不均衡"=w5677:dbl)
                    n2217 = call "输入分辨率计算-EV05.vi"("1字节?"=TRUE, "数值"=w5677, "偏移量"=0.0, "分辨率"=1.0) -> ("高字节1"=w5680:dbl)  [unwired: 1 in, 6 out]
                  }
                  frame Enabled {
                  }
                }
                n2218 = Build Array(w5676) -> (w5675:i32[])
              }
              frame 5 {
                # "单组电压不均衡"
                n2219 = disable-structure shown="启用" {
                  disable-tunnel: [w5692 w5695] -> w5687
                  disable-tunnel: [w5690 w5695] -> w5685
                  disable-tunnel: w5684 -> [w5689 _]
                  frame Disabled {
                    n2220 = Unbundle By Name(w5689) -> ("单组电压不均衡"=w5688:dbl)
                    n2221 = call "输入分辨率计算-EV05.vi"("1字节?"=FALSE, "数值"=w5688, "偏移量"=0.0, "分辨率"=0.001) -> ("低字节"=w5690:dbl, "高字节1"=w5692:dbl)  [unwired: 1 in, 5 out]
                  }
                  frame Enabled {
                    w5695 = 255 ("高字节1")
                  }
                }
                n2222 = Build Array(w5687, w5685) -> (w5686:i32[])
              }
              frame 6 {
                # "整组电压不均衡"
                n2223 = disable-structure shown="启用" {
                  disable-tunnel: [w5704 w5707] -> w5699
                  disable-tunnel: [w5702 w5707] -> w5697
                  disable-tunnel: w5696 -> [w5701 _]
                  frame Enabled {
                    n2224 = Unbundle By Name(w5701) -> ("整组电压不均衡"=w5700:dbl)
                    n2225 = call "输入分辨率计算-EV05.vi"("1字节?"=FALSE, "数值"=w5700, "偏移量"=0.0, "分辨率"=0.001) -> ("低字节"=w5702:dbl, "高字节1"=w5704:dbl)  [unwired: 1 in, 5 out]
                  }
                  frame Disabled {
                    w5707 = 255 ("高字节1")
                  }
                }
                n2226 = Build Array(w5699, w5697) -> (w5698:dbl[])
              }
              frame 7 {
                # "单体电压过高"
                n2227 = disable-structure shown="启用" {
                  disable-tunnel: [w5716 w5719] -> w5711
                  disable-tunnel: [w5714 w5719] -> w5709
                  disable-tunnel: w5708 -> [w5713 _]
                  frame Disabled {
                    n2228 = Unbundle By Name(w5713) -> ("单体电压过高"=w5712:dbl)
                    n2229 = call "输入分辨率计算-EV05.vi"("1字节?"=FALSE, "数值"=w5712, "偏移量"=0.0, "分辨率"=0.001) -> ("低字节"=w5714:dbl, "高字节1"=w5716:dbl)  [unwired: 1 in, 5 out]
                  }
                  frame Enabled {
                    w5719 = 255 ("高字节1")
                  }
                }
                n2230 = Build Array(w5711, w5709) -> (w5710:i32[])
              }
              frame 8 {
                # "单体电压过低"
                n2231 = disable-structure shown="启用" {
                  disable-tunnel: [w5728 w5731] -> w5723
                  disable-tunnel: [w5726 w5731] -> w5721
                  disable-tunnel: w5720 -> [w5725 _]
                  frame Disabled {
                    n2232 = Unbundle By Name(w5725) -> ("单体电压过低"=w5724:dbl)
                    n2233 = call "输入分辨率计算-EV05.vi"("1字节?"=FALSE, "数值"=w5724, "偏移量"=0.0, "分辨率"=0.001) -> ("低字节"=w5726:dbl, "高字节1"=w5728:dbl)  [unwired: 1 in, 5 out]
                  }
                  frame Enabled {
                    w5731 = 255 ("高字节1")
                  }
                }
                n2234 = Build Array(w5723, w5721) -> (w5722:i32[])
              }
              frame 9 {
                # "充电电流过高"
                n2235 = disable-structure shown="启用" {
                  disable-tunnel: [w5740 w5743] -> w5735
                  disable-tunnel: [w5738 w5743] -> w5733
                  disable-tunnel: w5732 -> [w5737 _]
                  frame Disabled {
                    n2236 = Unbundle By Name(w5737) -> ("充电电流过高"=w5736:dbl)
                    n2237 = call "输入分辨率计算-EV05.vi"("1字节?"=FALSE, "数值"=w5736, "偏移量"=-3000.0, "分辨率"=0.1) -> ("低字节"=w5738:dbl, "高字节1"=w5740:dbl)  [unwired: 1 in, 5 out]
                  }
                  frame Enabled {
                    w5743 = 255 ("高字节1")
                  }
                }
                n2238 = Build Array(w5735, w5733) -> (w5734:i32[])
              }
              frame 10 {
                # "放电电流过高"
                n2239 = disable-structure shown="启用" {
                  disable-tunnel: [w5752 w5755] -> w5747
                  disable-tunnel: [w5750 w5755] -> w5745
                  disable-tunnel: w5744 -> [w5749 _]
                  frame Disabled {
                    n2240 = Unbundle By Name(w5749) -> ("放电电流过高"=w5748:dbl)
                    n2241 = call "输入分辨率计算-EV05.vi"("1字节?"=FALSE, "数值"=w5748, "偏移量"=-3000.0, "分辨率"=0.1) -> ("低字节"=w5750:dbl, "高字节1"=w5752:dbl)  [unwired: 1 in, 5 out]
                  }
                  frame Enabled {
                    w5755 = 255 ("高字节1")
                  }
                }
                n2242 = Build Array(w5747, w5745) -> (w5746:i32[])
              }
              frame 11 {
                # "单组温度不均衡"
                n2243 = disable-structure shown="启用" {
                  disable-tunnel: [w5762 255 ("高字节1")] -> w5758
                  disable-tunnel: w5756 -> [w5760 _]
                  frame Disabled {
                    n2244 = Unbundle By Name(w5760) -> ("单组温度不均衡"=w5759:dbl)
                    n2245 = call "输入分辨率计算-EV05.vi"("1字节?"=TRUE, "数值"=w5759, "偏移量"=0.0, "分辨率"=1.0) -> ("高字节1"=w5762:dbl)  [unwired: 1 in, 6 out]
                  }
                  frame Enabled {
                  }
                }
                n2246 = Build Array(w5758) -> (w5757:i32[])
              }
              frame 12 {
                # "SOC过高"
                n2247 = Unbundle By Name(w5770) -> ("SOC过高"=w5769:dbl)
                n2248 = call "输入分辨率计算-EV05.vi"("1字节?"=FALSE, "数值"=w5769, "偏移量"=0.0, "分辨率"=0.1) -> ("低字节"=w5771:dbl, "高字节1"=w5772:dbl)  [unwired: 1 in, 5 out]
                n2249 = call "二进制解析-8.6.vi"("索引"=4, "数值"=w5772) -> ("低位子数组"=w5775:i32[])  [unwired: 3 out]
                n2250 = call "二进制解析-8.6.vi"("索引"=4, "数值"=w5771) -> ("低位子数组"=w5767:i32[], "高位子数组"=w5774:i32[])  [unwired: 2 out]
                n2251 = Insert Into Array(array=w5775, new element=w5774) -> (w5773:i32[])  [unwired: 1 in]
                n2252 = call "数值二进制转十进制-8.6.vi"("子数组"=w5773) -> ("十进制数值"=w5768:i32)  [unwired: 4 out]
                n2253 = disable-structure shown="启用" {
                  disable-tunnel: w5768 -> [w5783 _]
                  disable-tunnel: [w5783 255 ("高字节1")] -> w5766
                  disable-tunnel: [w5782 i32[] [] ("低位子数组 24")] -> _
                  disable-tunnel: w5767 -> [w5782 _]
                  frame Disabled {
                  }
                  frame Enabled {
                  }
                }
                n2254 = Build Array(w5766, w5766) -> (w5779:i32[])
              }
              frame 13 {
                # "SOC过低"
